vi "DSC_MonitorTask.vi"(1 "Task Trigger":refnum<class>, 2 "Task Destination":refnum<class>, 3 "Task Exception Event":refnum<class>, 5 "error in (no error)":errorcluster, 8 "timeout in ms (100)":i32=1000) -> (14 "Monitor TaskLoop":refnum<class "HGF_TaskLoop.lvclass">, 16 "Task Destination Event":refnum<class "HGF_Event.lvclass">, 17 "Task Trigger Event":refnum<class "HGF_Event.lvclass">, 18 "ExceptionTriggerEvent":refnum<class "HGF_TriggeredEvent.lvclass">, 19 "error out":errorcluster)   [LabVIEW 2012, in "HGF_DSC.lvlib" / "HGF_DSCMonitor.lvclass"]
doc: "VI creates TaskLoop with one Monitor Object.\n\nIf TaskTrigger is not a HGF_Event, a TaskQueue (timeout: input, standard Object: runMonitorVisitor) will be created.\nIf TaskDestination is not a HGF_Event, a TaskOccurrence (timeout: -1) will be created.\nIf TaskExceptionEvent is not a HGF_TriggerEvent, a TaskNotifier (timeout: 100) will be created.\n\nF.Berck@gsi.de\nGSI Darmstadt 2010"
uses:
  HGF_DSCMonitor.lvclass
  HGF_BaseClasses/HGF_TaskLoop/HGF_TaskLoop.lvclass
  HGF_BaseClasses/HGF_Event/HGF_Event.lvclass
  HGF_BaseClasses/HGF_TriggeredEvent/HGF_TriggeredEvent.lvclass
  HGF_DSCFactory/HGF_DSCFactory.lvclass
  HGF_SV/Visitors/HGF_SVMonitorVisitor/HGF_SVMonitorVisitor.lvclass
  HGF_BaseClasses/HGF_Notifier/HGF_Notifier.lvclass
  HGF_BaseClasses/HGF_TaskOnce/HGF_TaskOnce.lvclass
  HGF_BaseClasses/HGF_ThreadTask/HGF_ThreadTask.lvclass
  HGF_BaseClasses/HGF_Factory/HGF_Factory.lvclass
  HGF_BaseClasses/HGF_Queue/HGF_Queue.lvclass
  HGF_BaseClasses/HGF_Timing/HGF_Timing.lvclass
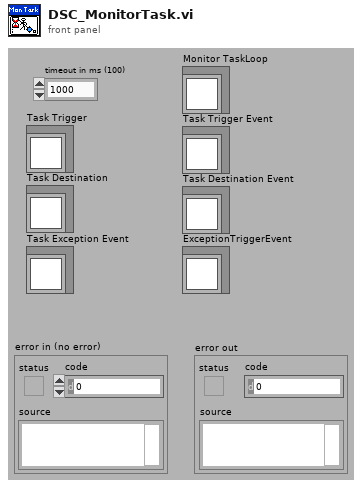
[diagram p1: front panel]
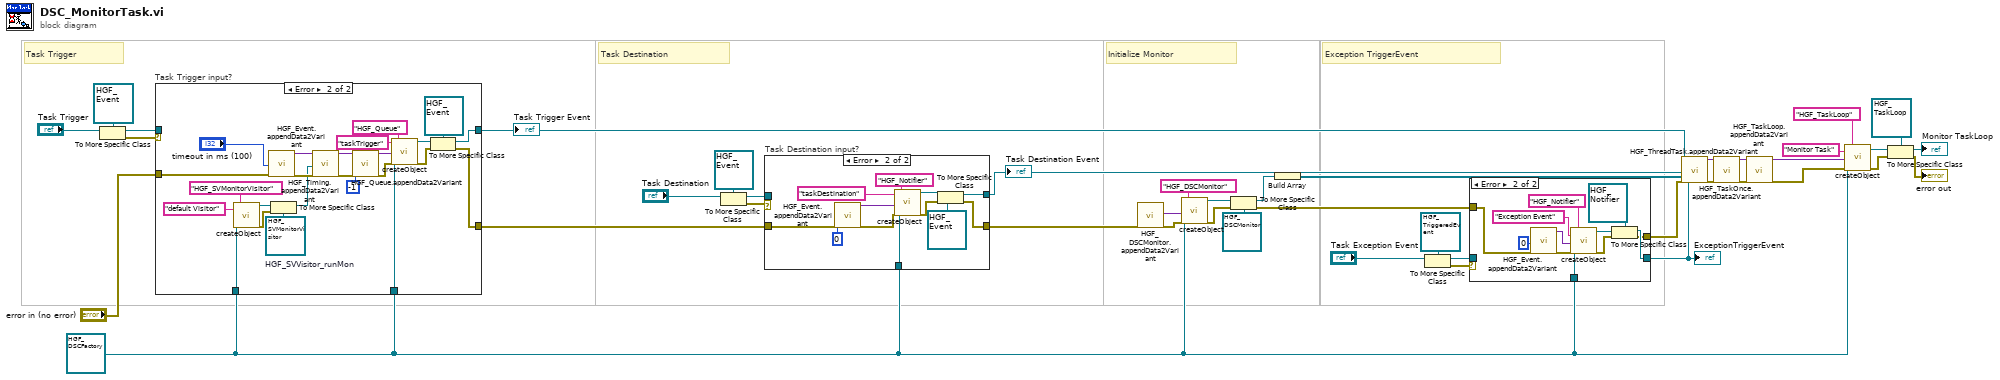
[diagram p0: block diagram]
diagram:
  w11 = refnum<class "HGF_DSCFactory.lvclass"> refnum ("DSC.lvlib:HGF_DSCFactory.lvclass")
  # "Exception TriggerEvent"
  # "Initialize Monitor"
  # "Task Destination"
  # "Task Trigger"
  n1 = To More Specific Class(target class=refnum<class "HGF_Event.lvclass"> refnum ("HGF_BaseClasses.lvlib:HGF_Event.lvclass"), reference="Task Trigger") -> (specific class reference=w13:refnum<class "HGF_Event.lvclass">, error out=w14:errorcluster)  [unwired: 1 in]
  n2 = case "Task Trigger input?" shown="Error" w14 {
    tunnel: w11 -> [_ w68]
    tunnel: [w44 w65] -> w12
    tunnel: [w43 w56] -> w7
    tunnel: "error in (no error)" -> [w43 w55]
    tunnel: w13 -> [w44 _]
    tunnel: w11 -> [_ w47]
    frame No Error {
    }
    frame Error {
      w46 = refnum<class "HGF_SVMonitorVisitor.lvclass"> refnum  # HGF_SVVisitor_runMon
      n3 = call "createObject.vi"("HGF_Factory"=w47, "objectName"="default Visitor", "className"="HGF_SVMonitorVisitor") -> ("HGF_Object"=w50:refnum<class "HGF_Factory.lvclass">, "error out"=w51:errorcluster)  [unwired: 14 in, 1 out]
      n4 = call "HGF_Event.appendData2Variant.vi"("timeout in ms (-1)"="timeout in ms (100)", "error in (no error)"=w55) -> ("dup initData"=w58:variant, "error out"=w57:errorcluster)  [unwired: 16 in]
      n5 = To More Specific Class(target class=w46, reference=w50, error in=w51) -> (specific class reference=w48:refnum<class "HGF_SVMonitorVisitor.lvclass">)  [unwired: 1 out]
      n6 = call "HGF_Timing.appendData2Variant.vi"("initData"=w58, "defaultObject"=w48, "error in (no error)"=w57) -> ("dup initData"=w61:variant, "error out"=w60:errorcluster)  [unwired: 15 in]
      n7 = call "HGF_Queue.appendData2Variant.vi"("initData"=w61, "maxQueueSize (-1)"=-1, "error in (no error)"=w60) -> ("dup initData"=w64:variant, "error out"=w63:errorcluster)  [unwired: 15 in]
      n8 = call "createObject.vi"("HGF_Factory"=w68, "objectName"="taskTrigger", "initializationData"=w64, "error in (no error)"=w63, "className"="HGF_Queue") -> ("HGF_Object"=w67:refnum<class "HGF_Factory.lvclass">, "error out"=w66:errorcluster)  [unwired: 12 in, 1 out]
      n9 = To More Specific Class(target class=refnum<class "HGF_Event.lvclass"> refnum ("HGF_BaseClasses.lvlib:HGF_Event.lvclass"), reference=w67, error in=w66) -> (specific class reference=w65:refnum<class "HGF_Event.lvclass">, error out=w56:errorcluster)
    }
  }
  "Task Trigger Event" <- w12
  n10 = To More Specific Class(target class=refnum<class "HGF_Event.lvclass"> refnum ("HGF_BaseClasses.lvlib:HGF_Event.lvclass"), reference="Task Destination") -> (specific class reference=w6:refnum<class "HGF_Event.lvclass">, error out=w8:errorcluster)  [unwired: 1 in]
  n11 = case "Task Destination input?" shown="Error" w8 {
    tunnel: [w70 w79] -> w27
    tunnel: [w69 w78] -> w26
    tunnel: w7 -> [w69 w75]
    tunnel: w11 -> [_ w72]
    tunnel: w6 -> [w70 _]
    frame No Error {
    }
    frame Error {
      n12 = call "HGF_Event.appendData2Variant.vi"("timeout in ms (-1)"=0, "error in (no error)"=w75) -> ("dup initData"=w77:variant, "error out"=w76:errorcluster)  [unwired: 16 in]
      n13 = call "createObject.vi"("HGF_Factory"=w72, "objectName"="taskDestination", "initializationData"=w77, "error in (no error)"=w76, "className"="HGF_Notifier") -> ("HGF_Object"=w81:refnum<class "HGF_Factory.lvclass">, "error out"=w80:errorcluster)  [unwired: 12 in, 1 out]
      n14 = To More Specific Class(target class=refnum<class "HGF_Event.lvclass"> refnum ("HGF_BaseClasses.lvlib:HGF_Event.lvclass"), reference=w81, error in=w80) -> (specific class reference=w79:refnum<class "HGF_Event.lvclass">, error out=w78:errorcluster)
    }
  }
  "Task Destination Event" <- w27
  n15 = call "HGF_DSCMonitor.appendData2Variant.vi"("error in (no error)"=w26) -> ("dup initData"=w34:variant, "error out"=w33:errorcluster)  [unwired: 17 in]
  n16 = call "createObject.vi"("HGF_Factory"=w11, "initializationData"=w34, "error in (no error)"=w33, "className"="HGF_DSCMonitor") -> ("HGF_Object"=w31:refnum<class "HGF_Factory.lvclass">, "error out"=w28:errorcluster)  [unwired: 13 in, 1 out]
  n17 = To More Specific Class(target class=refnum<class "HGF_DSCMonitor.lvclass"> refnum ("DSC.lvlib:HGF_DSCMonitor.lvclass"), reference=w31, error in=w28) -> (specific class reference=w30:refnum<class "HGF_DSCMonitor.lvclass">, error out=w24:errorcluster)
  n18 = Build Array(w30) -> (w32:refnum<class "HGF_DSCMonitor.lvclass">[])
  n19 = To More Specific Class(target class=refnum<class "HGF_TriggeredEvent.lvclass"> refnum ("HGF_BaseClasses.lvlib:HGF_TriggeredEvent.lvclass"), reference="Task Exception Event") -> (specific class reference=w3:refnum<class "HGF_TriggeredEvent.lvclass">, error out=w4:errorcluster)  [unwired: 1 in]
  n20 = case shown="Error" w4 {
    tunnel: [w84 w92] -> w2
    tunnel: [w83 w91] -> w25
    tunnel: w24 -> [w83 w90]
    tunnel: w11 -> [_ w85]
    tunnel: w3 -> [w84 _]
    frame No Error {
    }
    frame Error {
      n21 = call "HGF_Event.appendData2Variant.vi"("timeout in ms (-1)"=0, "error in (no error)"=w90) -> ("dup initData"=w88:variant, "error out"=w89:errorcluster)  [unwired: 16 in]
      n22 = call "createObject.vi"("HGF_Factory"=w85, "objectName"="Exception Event", "initializationData"=w88, "error in (no error)"=w89, "className"="HGF_Notifier") -> ("HGF_Object"=w95:refnum<class "HGF_Factory.lvclass">, "error out"=w94:errorcluster)  [unwired: 12 in, 1 out]
      n23 = To More Specific Class(target class=refnum<class "HGF_Notifier.lvclass"> refnum ("HGF_BaseClasses.lvlib:HGF_Notifier.lvclass"), reference=w95, error in=w94) -> (specific class reference=w92:refnum<class "HGF_Notifier.lvclass">, error out=w91:errorcluster)
    }
  }
  "ExceptionTriggerEvent" <- w2
  n24 = call "HGF_ThreadTask.appendData2Variant.vi"("taskTrigger"=w12, "taskDestination"=w27, "objectArray"=w32, "error in (no error)"=w25, "exceptionEvent"=w2) -> ("dup initData"=w42:variant, "error out"=w36:errorcluster)  [unwired: 13 in]
  n25 = call "HGF_TaskOnce.appendData2Variant.vi"("initData"=w42, "error in (no error)"=w36) -> ("dup initData"=w41:variant, "error out"=w37:errorcluster)  [unwired: 16 in]
  n26 = call "HGF_TaskLoop.appendData2Variant.vi"("initData"=w41, "error in (no error)"=w37) -> ("dup initData"=w19:variant, "error out"=w20:errorcluster)  [unwired: 16 in]
  n27 = call "createObject.vi"("HGF_Factory"=w11, "objectName"="Monitor Task", "initializationData"=w19, "error in (no error)"=w20, "className"="HGF_TaskLoop") -> ("HGF_Object"=w38:refnum<class "HGF_Factory.lvclass">, "error out"=w39:errorcluster)  [unwired: 12 in, 1 out]
  n28 = To More Specific Class(target class=refnum<class "HGF_TaskLoop.lvclass"> refnum ("HGF_BaseClasses.lvlib:HGF_TaskLoop.lvclass"), reference=w38, error in=w39) -> (specific class reference=→"Monitor TaskLoop":refnum<class "HGF_TaskLoop.lvclass">, error out=→"error out":errorcluster)
